vi "find_ergs.vi"(0 "VISA resource name":refnum<visa-resource-name>, 2 "Numeric":i32, 3 "error in (no error)":errorcluster) -> (5 "VISA resource name out":refnum<visa-resource-name>, 6 "unsigned byte array 2":u8[][](array[numeric]), 7 "error out":errorcluster)   [LabVIEW 2018]
panel:
  out "Errors?":bool
  out "Errors 2":bool
  out "Errors":bool
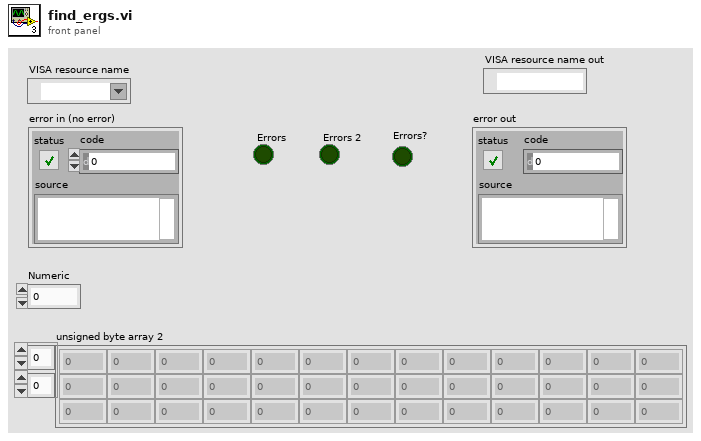
[diagram p1: front panel]
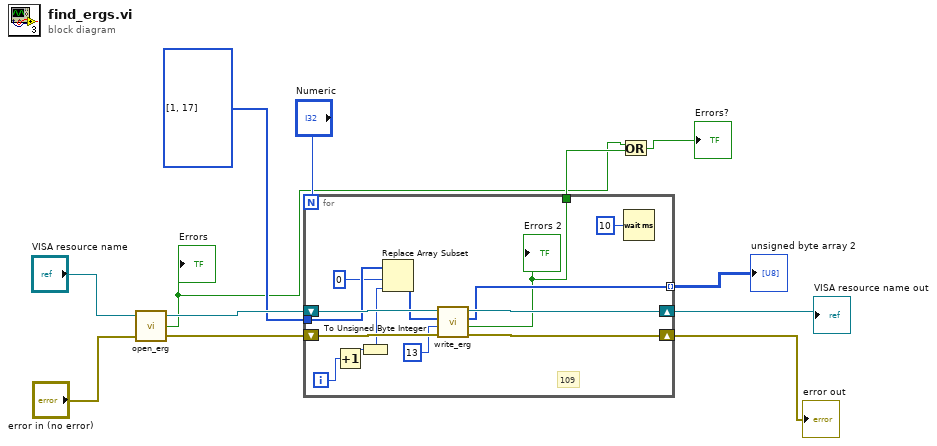
[diagram p0: block diagram]
diagram:
  n1 = call "open_erg.vi"("error in (no error)"="error in (no error)", "VISA resource name"="VISA resource name") -> ("error out"=w11:errorcluster, "Errors"=w1:bool, "VISA resource name out"=w12:refnum<visa-resource-name>)  [unwired: 1 in]
  "Errors" <- w1
  n2 = for {
    N: "Numeric" -> [_]
    tunnel: u8[] [1, 17] ("unsigned byte array") -> [w22]
    shift-right: [w24] -> w10
    shift-left: w12 -> [w26]
    shift-right: [w23] -> w4
    shift-left: w11 -> [w25]
    tunnel: [w19] -> w5 mode=indexing
    tunnel: [w13] -> w2
    i -> [w16]
    # "109"
    n3 = Increment(x=w16) -> (x+1=w15:i32)
    n4 = To Unsigned Byte Integer(number=w15) -> (unsigned 8bit integer=w17:u8)
    n5 = Replace Array Subset(array=w22, new element=w17, index=0) -> (w21:u8[])
    n6 = call "write_erg.vi"("error in (no error)"=w25, "byte count"=u32 13, "unsigned byte array"=w21, "VISA resource name"=w26) -> ("error out"=w23:errorcluster, "Errors"=w13:bool, "unsigned byte array 2"=w19:u8[], "VISA resource name out"=w24:refnum<visa-resource-name>)  [unwired: 4 in]
    "Errors 2" <- w13
    n7 = Wait (ms)(milliseconds to wait=u32 10) -> ()  [unwired: 1 out]
  }
  "unsigned byte array 2" <- w5
  "error out" <- w4
  "VISA resource name out" <- w10
  n8 = Or(x=w1, y=w2) -> (x .or. y?=→"Errors?":bool)
